vi "DTC.ValueCode.UpdateTable.vi"(8 "error in (no error)":errorcluster, 10 "DTC Codes":refnum<vi>, 11 "Device Item Ref in":T1 format="%.0x") -> (0 "error out":errorcluster, 3 "Device Item Ref out":T1=18446744073709551615 format="%.0x")   [LabVIEW 2019, in "Diagnostics Addon System Explorer.lvlib"]
uses:
  Diagnostics Addon System Explorer.lvlib
  <vilib>/NI VeriStand/Custom Device API/Custom Device Item Ref.ctl
  Types/FG.Action.ctl
  Addon Shared/SubVIs/Constants.vi
  <vilib>/NI/NI VeriStand Advanced SysDef API/SysDef API/SysDef.Property.Set.vi
  <vilib>/NI/NI VeriStand Advanced SysDef API/_SubVIs/SysDef.Property.Set.I32.vi
  <vilib>/NI/NI VeriStand Advanced SysDef API/_SubVIs/SysDef.Property.Set.U32.vi
  <vilib>/NI/NI VeriStand Advanced SysDef API/_SubVIs/SysDef.Property.Set.DBL.Array.vi
  <vilib>/NI/NI VeriStand Advanced SysDef API/_SubVIs/SysDef.Property.Set.String.Array.vi
  <vilib>/NI VeriStand/Custom Device API/NI VeriStand - Get Item Property.vi
  <vilib>/NI VeriStand/Custom Device API/Get Item Property (I32).vi
  <vilib>/NI VeriStand/Custom Device API/Get Item Property (U32).vi
  <vilib>/NI VeriStand/Custom Device API/Get Item Property (Double Array).vi
  <vilib>/NI VeriStand/Custom Device API/Get Item Property (String Array).vi
  <vilib>/NI VeriStand/Custom Device API/Custom Device API.lvlib
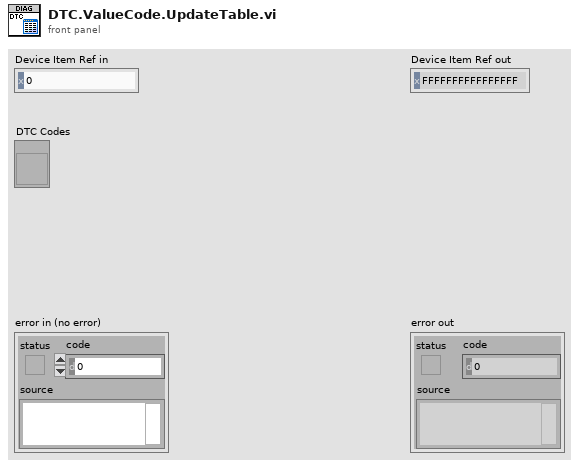
[diagram p1: front panel]
types:
  T1 = typedef "Custom Device API.lvlib/Custom Device Item Ref.ctl" = u64
  T2 = typedef "Diagnostics Addon System Explorer.lvlib/FG.Action.ctl" = enum16{"Get", "Set"}
  T3 = typedef "Diagnostics Addon Shared.lvlib/DTC.Settings.ctl" = cluster{"Descriptor":T4, "Value.Code":dbl[], "Value.String":string[], "Value.J2012String":string[], "Status.Code":dbl[], "Status.String":string[]}
  T4 = typedef "Diagnostics Addon Shared.lvlib/DTC.Descriptor.ctl" = cluster{"DTC Byte Length":i32, "Status Byte Length":i32, "Add Data Byte Length":i32, "Byte Order":enum16{"Motorola", "Intel"}}
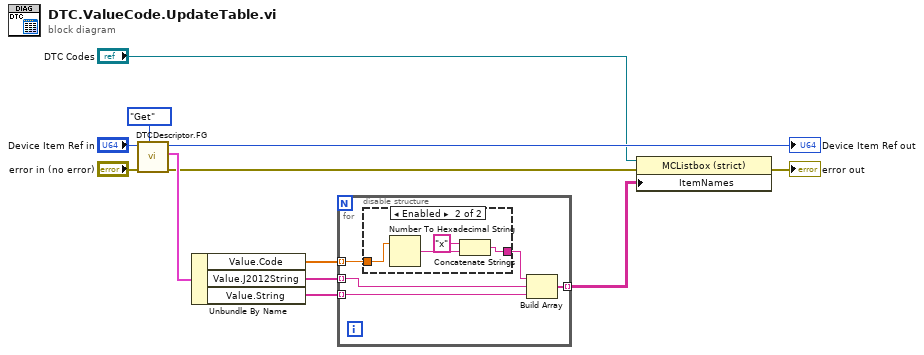
[diagram p0: block diagram]
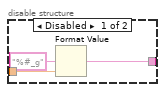
[diagram p2: hidden frame]
diagram:
  n1 = call "DTCDescriptor.FG.vi"("Action"=FG.Action."Get", "error in (no error)"="error in (no error)", "Device Item Ref in"="Device Item Ref in") -> ("error out"=w7:errorcluster, "DTC descriptor"=w8:T3, "Device Item Ref out"=→"Device Item Ref out":T1)  [unwired: 6 in]
  n2 = Unbundle By Name(w8) -> ("Value.Code"=w5:dbl[], "Value.J2012String"=w1:string[], "Value.String"=w4:string[])
  n3 = for {
    tunnel: w5 -> [w17] mode=indexing
    tunnel: w4 -> [w15] mode=indexing
    tunnel: [w14] -> w3 mode=indexing
    tunnel: w1 -> [w13] mode=indexing
    n4 = disable-structure shown="Enabled" {
      disable-tunnel: w17 -> [w20 w23]
      disable-tunnel: [w18 w22] -> w16
      frame Disabled {
        n5 = Format Value(format string="%#_g", value (0)=w20) -> (output string=w18:string)  [unwired: 1 in]
      }
      frame Enabled {
        n6 = Number To Hexadecimal String(2:w23) -> (0:w24:string)  [unwired: 1 in]
        n7 = Concatenate Strings("x" ("string"), w24) -> (w22:string)
      }
    }
    n8 = Build Array(w16, w13, w15) -> (w14:string[])
  }
  n9 = property class="MCListbox (strict)"(reference="DTC Codes", error in=w7, "ItemNames"=w3) -> (error out=→"error out":errorcluster)  [unwired: 1 out]
